vi "CollectISEOnly.vi"() -> ()   [LabVIEW 2016]
uses:
  <vilib>/Platform/TimedLoop/XDataNode/timing_clust.ctl
  <vilib>/Platform/TimedLoop/XDataNode/nitl_modes.ctl
  <vilib>/Platform/TimedLoop/XDataNode/wakeup.ctl
  <vilib>/Analysis/baseanly.llb/Mean (DBL).vi
  <vilib>/Utility/file.llb/Write Delimited Spreadsheet (string).vi
  <vilib>/Platform/TimedLoop/XDataNode/loadnilvce.vi
  <vilib>/Utility/file.llb/Write Delimited Spreadsheet (DBL).vi
  <vilib>/Platform/TimedLoop/XDataNode/XDataNode.xnode
  <resource>/objmgr/ni.var.rc
  <vilib>/Platform/TimedLoop/XDataNode/XDNodeRunTimeDep.lvlib
  <vilib>/Analysis/NI_AALBase.lvlib
panel:
  in  "Buffer Size":i32=100
  out "Saving?":bool
  out "NH4 Probe":refnum<k21>="ni.var.io://localhost/Mod6/AI0"
  out "Na Probe":refnum<k21>="ni.var.io://localhost/Mod6/AI1"
  out "new file path (Not A Path if cancelled)":path
  in  "File Name:":string
  out "Headers":string[](array[string])
  out "error out":errorcluster
  out "String 6":string="Na"
  out "NH4 Live":dbl format="%#_4g"
  out "Na Live":dbl format="%#_4g"
  out "current sample":dbl format="%#_3g"
  out "Date":string="K"
  out "Time":string="K"
  out "iter number":i32
  in  "stop":bool
  out "All data":dbl[][](array[numeric]) format="%#3.4f"
  in  "error in":errorcluster
  out "String 2":string="NH4"
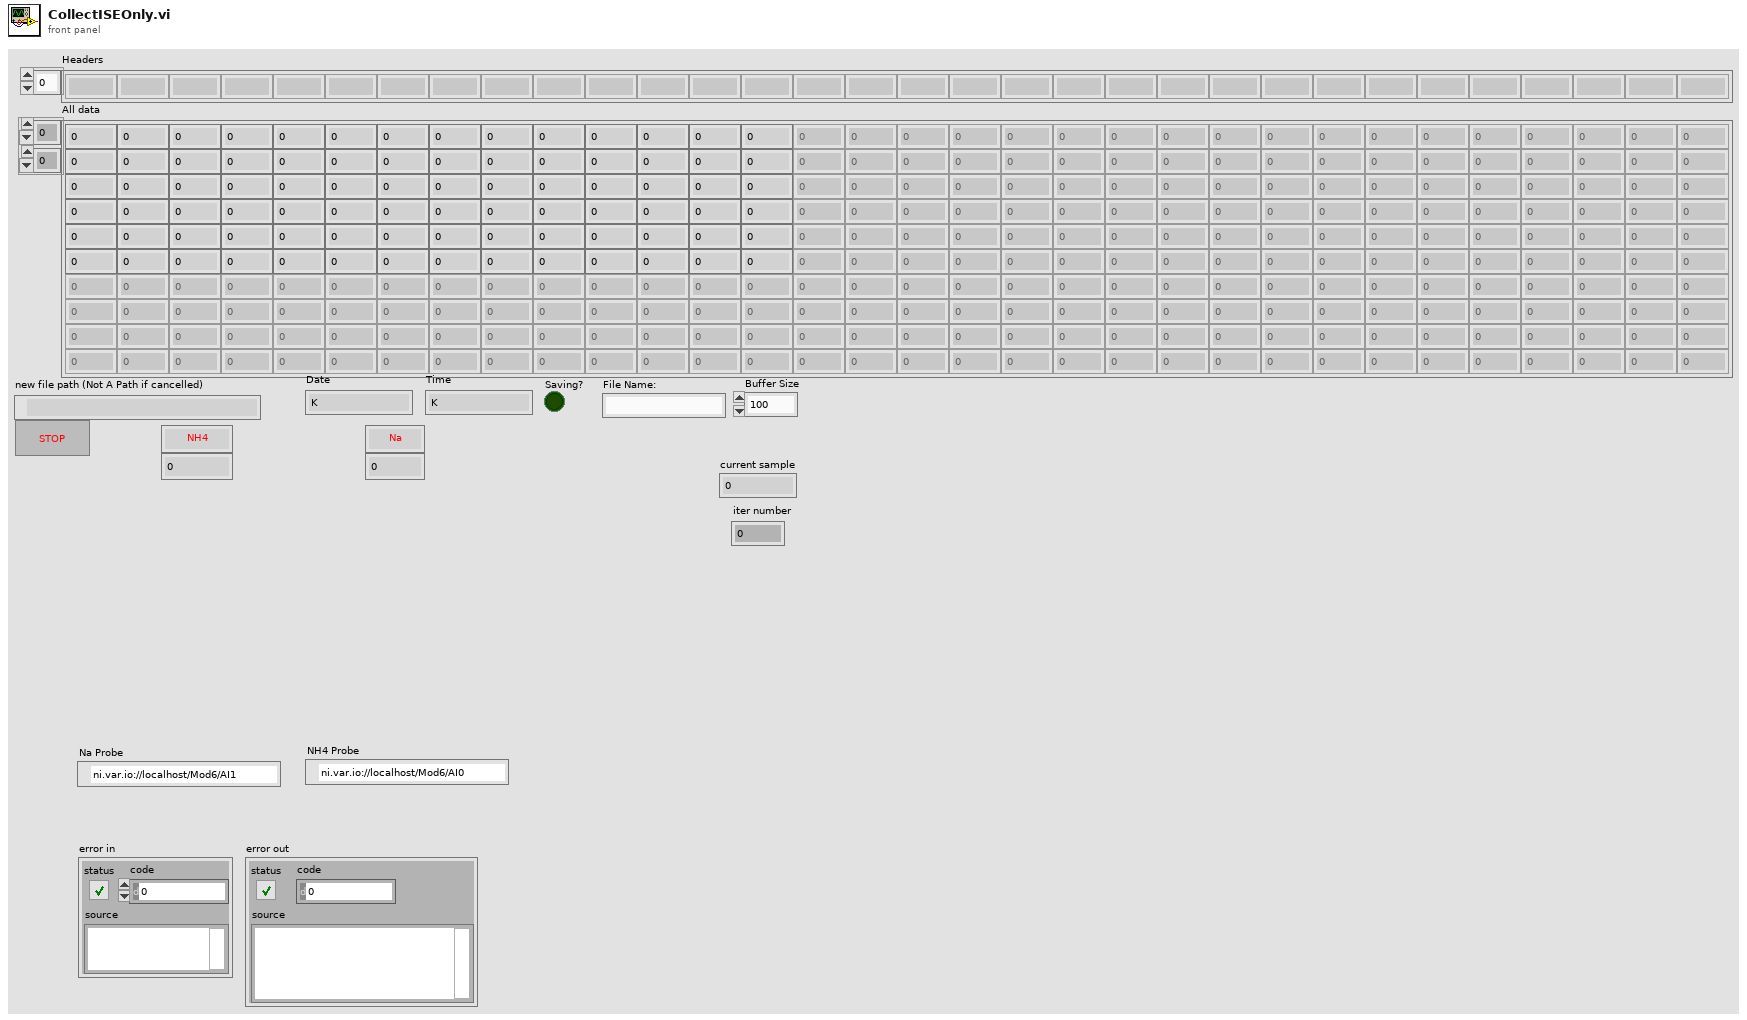
[diagram p1: front panel]
types:
  T1 = typedef "XDNodeRunTimeDep.lvlib/timing_clust.ctl" = cluster{"Expected End [f-1]":u64, "Actual End [f-1]":u64, "Finished Late? [f-1]":bool, "Expected End [i-1]":u64, "Actual End [i-1]":u64, "Finished Late? [i-1]":bool, "Expected Start [i]":u64, "Actual Start [i]":u64, "Expected Start [f]":u64, "Actual Start [f]":u64, "Source Name":string, "Structure Name":string, "Period":i64, "Deadline":i64, "Offset":i64, "Start":i64, "Priority":i32, "Timeout":i32, "Mode":T2, "Wakeup Reason":T3, "Error":errorcluster, "Source Type":string, "Secondary Source Type":string, "Global End Time":u64, "Global Start Time":u64, "Frame Duration":u64, "Iteration Duration":u64, "Assigned CPU":i32, "I/O Scan Engine Mode":u32}
  T2 = typedef "XDNodeRunTimeDep.lvlib/nitl_modes.ctl" = enum32{"No Change", "Process missed periods, maintain original phase", "Discard missed periods, maintain original phase", "Process missed periods, ignore original phase", "Discard missed periods, ignore original phase"}
  T3 = typedef "XDNodeRunTimeDep.lvlib/wakeup.ctl" = enum32{"Normal", "Aborted", "Asynchronous wakeup", "Timing source error", "Timed loop error", "Timeout"}
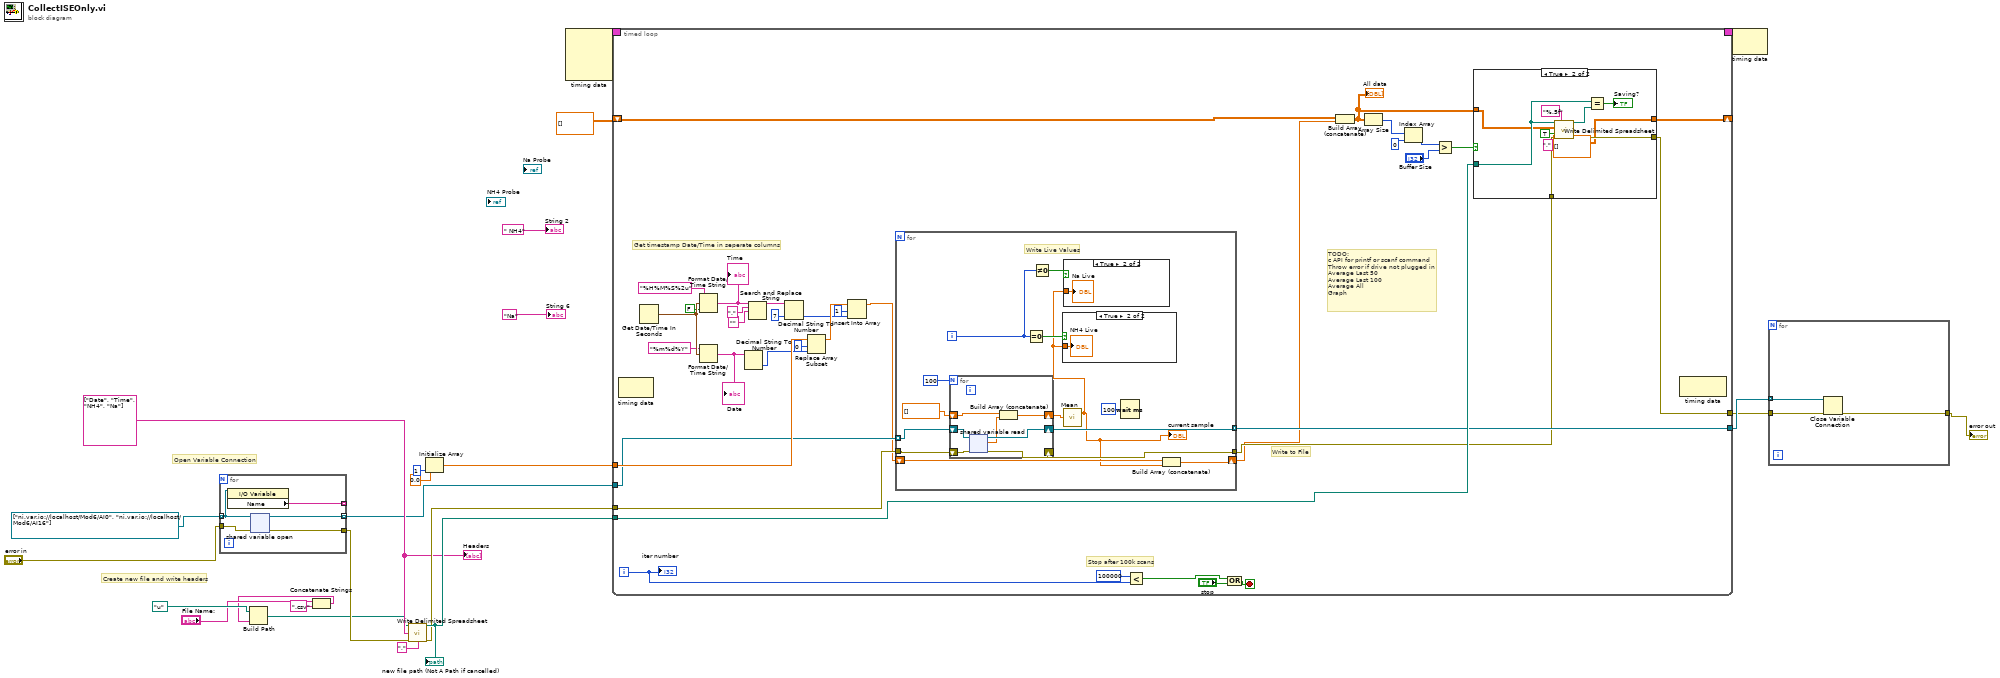
[diagram p0: block diagram]
diagram:
  w13 = string[] ["Date", "Time", "NH4", "Na"]
  # "Create new file and write headers"
  # "Open Variable Connection"
  n1 = for {
    tunnel: refnum<k21>[] ["ni.var.io://localhost/Mod6/AI0", "ni.var.io://localhost/Mod6/AI16"] -> [w26] mode=indexing
    tunnel: "error in" -> [w29]
    tunnel: [w28] -> w10 mode=indexing
    tunnel: [w27] -> w6
    tunnel: [w25] -> _ mode=indexing
    n2 = property class="I/O Variable"(reference=w26) -> ("Name"=w25:string)  [unwired: 1 in, 2 out]
    n3 = shared-variable-open(w26, w29) -> (w28:refnum<k21>, w27:errorcluster)  [unwired: 1 in]
  }
  n4 = Concatenate Strings("File Name:", ".csv" ("string")) -> (w7:string)
  n5 = Build Path(base path=path "u:/" ("Save to:"), name or relative path=w7) -> (appended path=w5:path)
  n6 = call-poly <vilib>:"Write Delimited Spreadsheet.vi"("file path (dialog if empty)"=w5, "1D data"=w13, "error in (no error)"=w6, "delimiter (\\t)"="," ("delimiter (\\t)")) -> ("new file path (Not A Path if cancelled)"=w20:path, "error out"=w18:errorcluster)  [unwired: 10 in]
  "new file path (Not A Path if cancelled)" <- w20
  n7 = Initialize Array(0.0 ("element"), 1 ("dimension size")) -> (w21:dbl[])
  n8 = node-c288() -> (w24:T1)  [unwired: 4 in]
  n9 = timed-loop {
    timing: w24 -> [_]
    timing-out: [_] -> w23
    tunnel: w21 -> [w56]
    tunnel: w18 -> [w66]
    tunnel: w20 -> [w39]
    shift-right: [w38] -> _
    shift-left: dbl[][] [] -> [w49]
    tunnel: w10 -> [w33]
    tunnel: [w36] -> w4
    tunnel: [w34] -> w3
    i -> [w50]
    stop <- w52 stop-if-true
    # "TODO: \nc API for printf or scanf command\nThrow error if drive not plugged in\nAverage Last 50\nAverage Last 100\nAverage All\nGraph"
    # "Stop after 100k scans"
    # "Write to File"
    # "Get timestamp Date/Time in seperate columns"
    n10 = node-c288() -> ()  [unwired: 1 in, 1 out]
    n11 = Get Date/Time In Seconds() -> (seconds since 1Jan1904=w64:timestamp)
    n12 = Format Date/Time String(time format string (%c)="%H%M%S%2u", seconds (now)=w64, UTC format=FALSE) -> (date/time string=w60:string)
    "Time" <- w60
    n13 = Format Date/Time String(time format string (%c)="%m%d%Y", seconds (now)=w64) -> (date/time string=w47:string)  [unwired: 1 in]
    "Date" <- w47
    n14 = Decimal String To Number(string=w47) -> (number=w46:i32)  [unwired: 2 in, 1 out]
    n15 = Search and Replace String(input string=w60, search string=".", replace string="") -> (result string=w59:string)  [unwired: 5 in, 3 out]
    n16 = Decimal String To Number(string=w59, default (0L)=7) -> (number=w45:i32)  [unwired: 1 in, 1 out]
    n17 = Replace Array Subset(array=w56, new element=w46, index=0) -> (w55:dbl[])
    n18 = Insert Into Array(array=w55, index=1, new element=w45) -> (w32:dbl[])
    n19 = for {
      tunnel: w66 -> [w92]
      shift-right: [w84] -> w31
      shift-left: w32 -> [w83]
      tunnel: [w87] -> w35
      tunnel: w33 -> [w86] mode=indexing
      tunnel: [w85] -> w36 mode=indexing
      i -> [w89]
      # "Write Live Values"
      n20 = for {
        N: 100 ("sample length") -> [_]
        shift-right: [w98] -> w87
        shift-left: w92 -> [w99]
        shift-right: [w96] -> w85
        shift-left: w86 -> [w97]
        shift-right: [w94] -> w81
        shift-left: dbl[] [] -> [w93]
        n21 = shared-variable-read(w97, w99) -> (w96:refnum<k21>, w98:errorcluster, w95:dbl)  [unwired: 1 out]
        n22 = Build Array (concatenate)(w93, w95) -> (w94:dbl[])
      }
      n23 = Equal To 0?(x=w89) -> (x = 0?=w90:bool)
      n24 = Not Equal To 0?(x=w89) -> (x != 0?=w91:bool)
      n25 = call-poly <vilib>:"Mean.vi"("X"=w81) -> ("mean"=w80:dbl)  [unwired: 1 out]
      "current sample" <- w80
      n26 = case shown="True" w90 {
        tunnel: w80 -> [_ w101]
        frame False {
        }
        frame True {
          "NH4 Live" <- w101
        }
      }
      n27 = case shown="True" w91 {
        tunnel: w80 -> [_ w100]
        frame False {
        }
        frame True {
          "Na Live" <- w100
        }
      }
      n28 = Wait (ms)(milliseconds to wait=u32 100) -> ()  [unwired: 1 out]
      n29 = Build Array (concatenate)(w83, w80) -> (w84:dbl[])
    }
    n30 = Less?(x=100000, y=w50) -> (x < y?=w51:bool)
    n31 = Compound Arithmetic op=OR(w51, "stop") -> (w52:bool)
    n32 = Build Array (concatenate)(w49, w31) -> (w37:dbl[][])
    "All data" <- w37
    n33 = Array Size(array=w37) -> (size(s)=w43:i32[])
    n34 = Index Array(array=w43, index=0) -> (element=w41:i32)
    n35 = Greater?(x=w41, y="Buffer Size") -> (0:w40:bool)
    n36 = case shown="True" w40 {
      tunnel: w37 -> [w67 w75]
      tunnel: w39 -> [_ w76]
      tunnel: [w67 dbl[][] []] -> w38
      tunnel: w35 -> [w68 w74]
      tunnel: [w68 w73] -> w34
      frame False {
      }
      frame True {
        n37 = call-poly <vilib>:"Write Delimited Spreadsheet.vi"("file path (dialog if empty)"=w76, "format (%.3f)"="%.5f", "2D data"=w75, "append to file? (new file:F)"=TRUE, "error in (no error)"=w74, "delimiter (\\t)"="," ("delimiter (\\t)")) -> ("new file path (Not A Path if cancelled)"=w77:path, "error out"=w73:errorcluster)  [unwired: 8 in]
        n38 = Equal?(x=w76, y=w77) -> (x = y?=→"Saving?":bool)
      }
    }
    n39 = node-c288() -> ()  [unwired: 1 in, 1 out]
    "iter number" <- w50
  }
  n40 = node-c288(w23) -> ()  [unwired: 1 out]
  n41 = for {
    tunnel: [w106] -> w17
    tunnel: w4 -> [w105] mode=indexing
    tunnel: w3 -> [w104]
    n42 = Close Variable Connection(8:w104, 11:w105) -> (0:w106:errorcluster)
  }
  "error out" <- w17
  "String 2" <- " NH4"
  "String 6" <- "Na"
  "Headers" <- w13
